vi "Close Device Core.vi"(8 "error in (no error)":errorcluster, 11 "CS++PPG in":refnum<class "CS++PPG.lvclass">) -> (0 "error out":errorcluster, 3 "CS++PPG out":refnum<class "CS++PPG.lvclass">)   [LabVIEW 2015, in "CS++PPG.lvlib" / "CS++PPG.lvclass"]
doc: "Close device driver connection."
uses:
  CS++PPG.lvclass
  CSPP_Core/Actors/CS++DeviceActor/CS++DeviceActor.lvclass
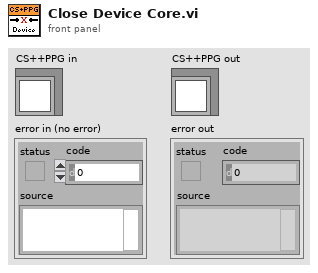
[diagram p1: front panel]
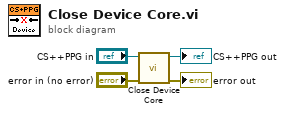
[diagram p0: block diagram]
diagram:
  n1 = call-parent "Close Device Core.vi"("error in (no error)"="error in (no error)", "CS++DeviceActor in"="CS++PPG in") -> ("error out"=→"error out":errorcluster, "CS++DeviceActor out"=→"CS++PPG out":refnum<class "CS++PPG.lvclass">)  [unwired: 8 in]
